vi "SendItemSelectedEvent.vi"(8 "error in (no error)":errorcluster, 10 "ProjectItem":refnum<vi>, 11 "_LVCMPlugin in":refnum<class "GCMPlugin.lvclass">) -> (0 "error out":errorcluster, 3 "_LVCMPlugin out":refnum<class "GCMPlugin.lvclass">)   [LabVIEW 2014, in "GCMPlugin.lvclass"]
uses:
  GCMPlugin/GCMPlugin.lvclass
  GCMPlugin/GCMPlugin.lvclass/GCMPlugin.ctl
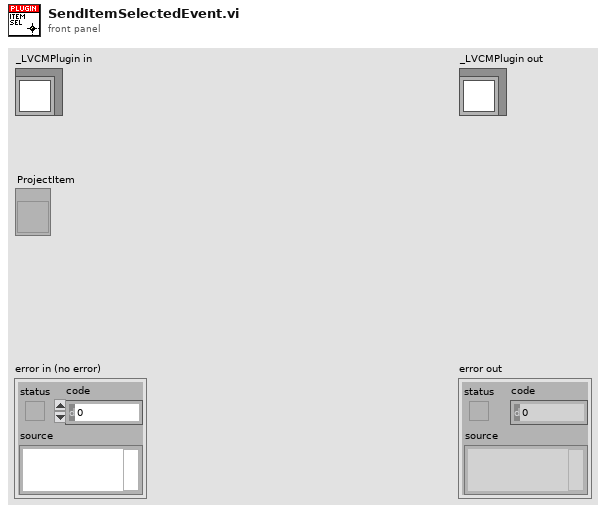
[diagram p1: front panel]
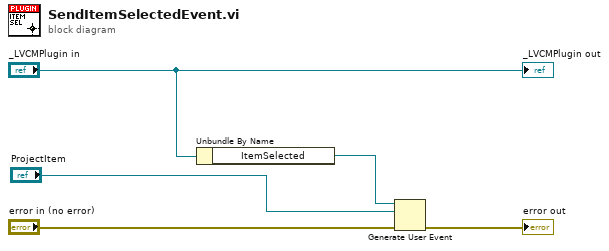
[diagram p0: block diagram]
diagram:
  n1 = Unbundle By Name("_LVCMPlugin in") -> ("ItemSelected"=w1:refnum<user-event>)
  n2 = Generate User Event(user event=w1, event data cluster="ProjectItem", error in="error in (no error)") -> (error out=→"error out":errorcluster)  [unwired: 1 in, 1 out]
  "_LVCMPlugin out" <- "_LVCMPlugin in"
